vi "Create All Message Queues.vi"(8 "error in (no error)":errorcluster) -> (0 "error out":errorcluster, 3 "Message Queues out":T1)   [LabVIEW 2024, in "Message Queue.lvlib"]
doc: "This VI creates and initializes all the message queues for your application. If your application requires more than one message queue, right-click the \"Message Queues\" constant above and select Open Type Def. Add the new Message Queue(s) to the type definition, then initialize them in this VI."
uses:
  Message Queue.lvlib
  All Message Queues.ctl
  Message Cluster.ctl
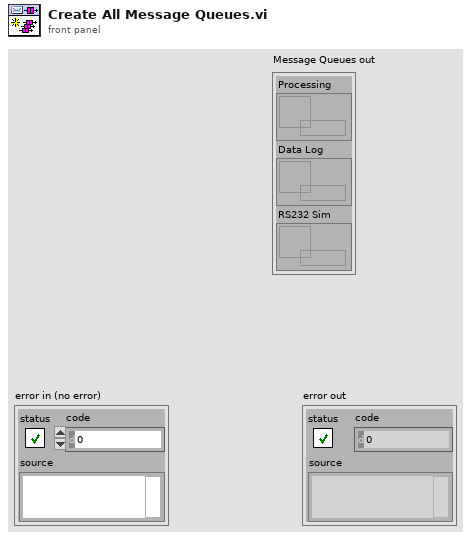
[diagram p1: front panel]
types:
  T1 = typedef "Message Queue.lvlib/All Message Queues.ctl" = cluster{"Processing":refnum<queue>, "Data Log":refnum<queue>, "RS232 Sim":refnum<queue>}
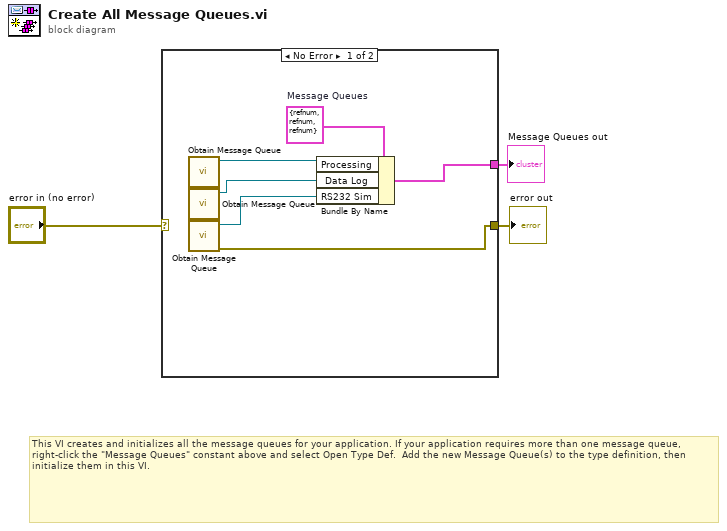
[diagram p0: block diagram]
diagram:
  # "This VI creates and initializes all the message queues for your application. If your application requires more than one message queue, right-click the \"Message Queues\" constant above and select Open Type Def.  Add the new Message Queue(s) to the type definition, then initialize them in this VI."
  n1 = case shown="No Error" "error in (no error)" {
    selector: "error in (no error)" -> [_ w10]
    tunnel: [w4 w10] -> w3
    tunnel: [w8 _] -> w2
    frame No Error {
      w9 = T1 {"Processing"=refnum, "Data Log"=refnum, "RS232 Sim"=refnum}  # Message Queues
      n2 = call "Obtain Message Queue.vi"() -> ("Message Queue"=w7:refnum<queue>)  [unwired: 10 in, 1 out]
      n3 = call "Obtain Message Queue.vi"() -> ("Message Queue"=w6:refnum<queue>)  [unwired: 10 in, 1 out]
      n4 = call "Obtain Message Queue.vi"() -> ("error out"=w4:errorcluster, "Message Queue"=w5:refnum<queue>)  [unwired: 10 in]
      n5 = Bundle By Name(cluster=w9, "Processing"=w7, "Data Log"=w6, "RS232 Sim"=w5) -> (w8:T1)
    }
    frame Error {
    }
  }
  "Message Queues out" <- w2
  "error out" <- w3
